vi "server send and receive data .vi"(8 "error in (no error)":errorcluster, 10 "Option":T1, 11 "Data in":i32[](array[numeric])) -> (0 "error out":errorcluster, 3 "Data out":i32[](array[numeric]))   [LabVIEW 2020, in "tcp ip server.lvclass"]
uses:
  tcp ip server.lvclass
  Controls/TCP IP FGV Option Control.ctl
  tcp ip server.lvclass/tcp ip server.ctl
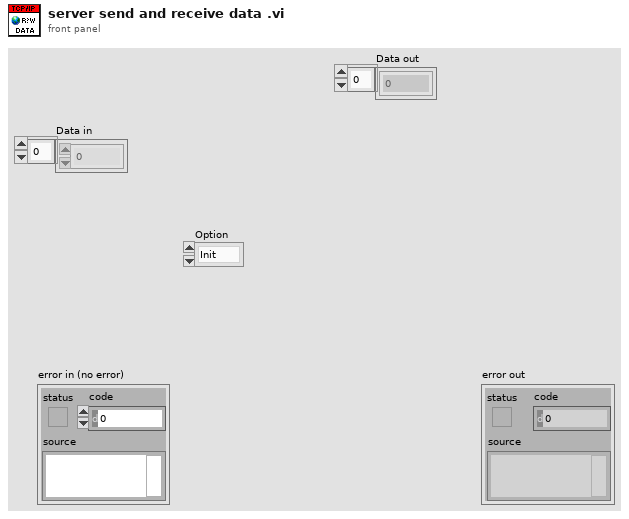
[diagram p1: front panel]
types:
  T1 = typedef "TCP IP FGV Option Control.ctl" = enum16{"Init", "Read Server Data", "Write Client Data", "Read Client Data", "Write Server Data"}
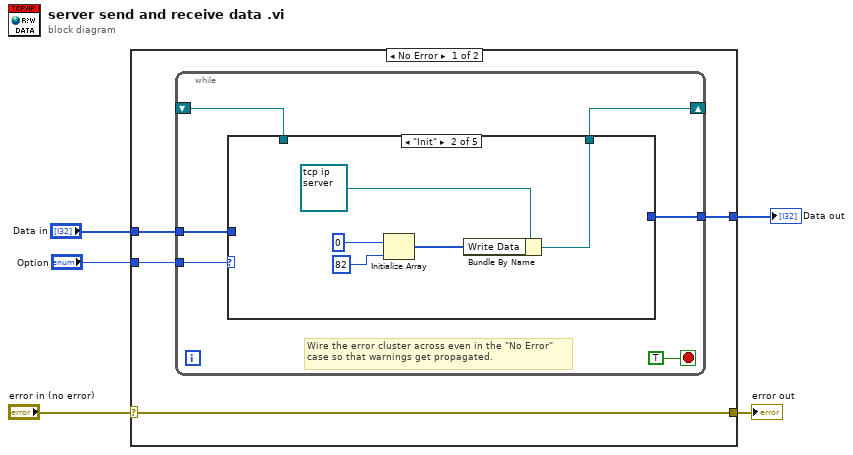
[diagram p0: block diagram]
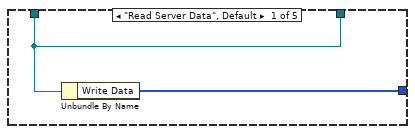
[diagram p2: hidden frame]
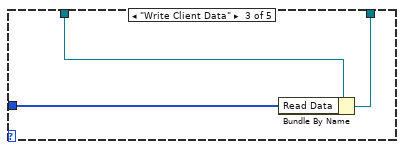
[diagram p3: hidden frame]
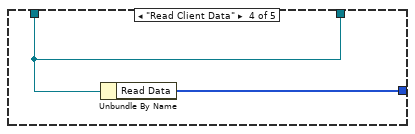
[diagram p4: hidden frame]
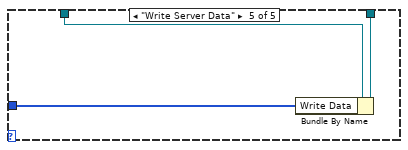
[diagram p5: hidden frame]
diagram:
  n1 = case shown="No Error" "error in (no error)" {
    selector: "error in (no error)" -> [w9 w31]
    tunnel: [w9 w31] -> w4
    tunnel: "Option" -> [w8 _]
    tunnel: [w7 _] -> w2
    tunnel: "Data in" -> [w6 _]
    frame No Error {
      n2 = while {
        tunnel: w8 -> [w15]
        shift-right: [w13] -> _
        shift-left: _ -> [w14]
        tunnel: [w11] -> w7
        tunnel: w6 -> [w10]
        stop <- TRUE stop-if-true
        # "Wire the error cluster across even in the \"No Error\"\ncase so that warnings get propagated."
        n3 = case shown="\"Init\"" w15 {
          tunnel: w14 -> [w17 _ w25 w27 w30]
          tunnel: [w17 w21 w24 w27 w29] -> w13
          tunnel: [w16 _ _ w26 _] -> w11
          tunnel: w10 -> [_ _ w23 _ w28]
          frame "Read Server Data", Default {
            n4 = Unbundle By Name(w17) -> ("Write Data"=w16:i32[])
          }
          frame "Init" {
            n5 = Initialize Array(0 ("Numeric"), 82 ("dimension size")) -> (w19:i32[])
            n6 = Bundle By Name(cluster=refnum<class "tcp ip server.lvclass"> refnum ("tcp ip server in"), "Write Data"=w19) -> (w21:refnum<class "tcp ip server.lvclass">)
          }
          frame "Write Client Data" {
            n7 = Bundle By Name(cluster=w25, "Read Data"=w23) -> (w24:refnum<class "tcp ip server.lvclass">)
          }
          frame "Read Client Data" {
            n8 = Unbundle By Name(w27) -> ("Read Data"=w26:i32[])
          }
          frame "Write Server Data" {
            n9 = Bundle By Name(cluster=w30, "Write Data"=w28) -> (w29:refnum<class "tcp ip server.lvclass">)
          }
        }
      }
    }
    frame Error {
    }
  }
  "error out" <- w4
  "Data out" <- w2
